vi "Extract Coefs for Network.vi"(9 "Min Array":dbl[](array[numeric]), 11 "Max Array":dbl[](array[numeric])) -> (1 "Y Scaling Vector":dbl[](array[numeric]), 3 "X Scaling Vector":dbl[](array[numeric]))   [LabVIEW 2013, in "Super Simple Neural Network.lvlib"]
uses:
  Super Simple Neural Network.lvlib
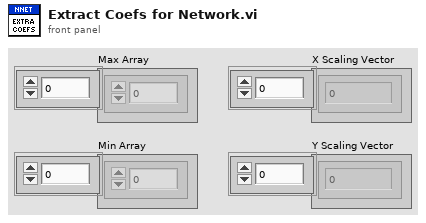
[diagram p1: front panel]
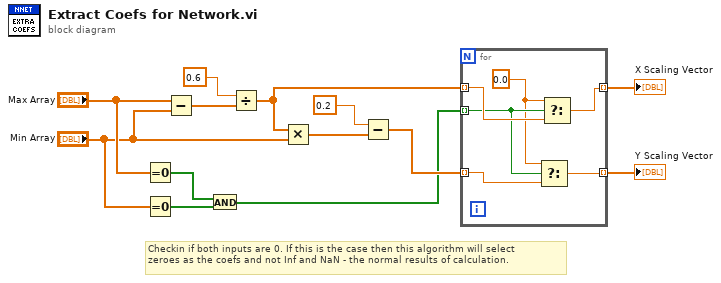
[diagram p0: block diagram]
diagram:
  # "Checkin if both inputs are 0. If this is the case then this algorithm will select\nzeroes as the coefs and not Inf and NaN - the normal results of calculation."
  n1 = Equal To 0?(x="Max Array") -> (x = 0?=w6:bool[])
  n2 = Equal To 0?(x="Min Array") -> (x = 0?=w7:bool[])
  n3 = Subtract(x="Max Array", y="Min Array") -> (x-y=w12:dbl[])
  n4 = And(x=w6, y=w7) -> (x .and. y?=w1:bool[])
  n5 = Divide(x=0.6, y=w12) -> (x/y=w3:dbl[])
  n6 = Multiply(x=w3, y="Min Array") -> (x*y=w10:dbl[])
  n7 = Subtract(x=0.2, y=w10) -> (x-y=w4:dbl[])
  n8 = for {
    tunnel: [w16] -> w5 mode=indexing
    tunnel: w4 -> [w17] mode=indexing
    tunnel: w3 -> [w19] mode=indexing
    tunnel: [w18] -> w2 mode=indexing
    tunnel: w1 -> [w15] mode=indexing
    w14 = 0.0 ("t")
    n9 = Select(t=w14, s=w15, f=w17) -> (s? t:f=w16:dbl)
    n10 = Select(t=w14, s=w15, f=w19) -> (s? t:f=w18:dbl)
  }
  "X Scaling Vector" <- w2
  "Y Scaling Vector" <- w5
